vi "IR measure read.vi"(8 "error in (no error)":errorcluster, 11 "ref array":refnum<class "IR sensor.lvclass">[](array[class])) -> (0 "error out":errorcluster, 4 "output cluster":T1, 5 "Waveform Chart":T2(graph))   [LabVIEW 2019]
uses:
  IR out.ctl
  FPGA_subVIs/low level/IR sensor/IR sensor.lvclass
  <vilib>/ptbypt/NI_PtbyPt.lvlib
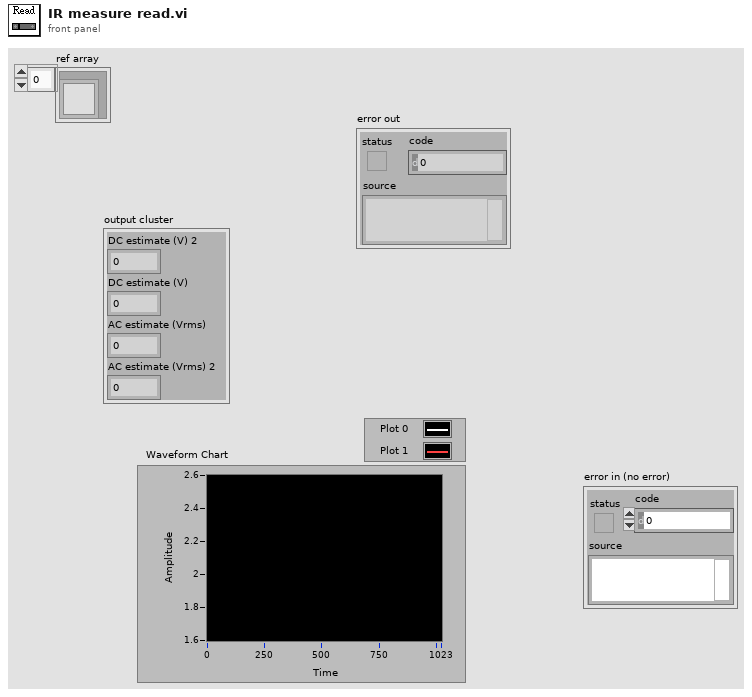
[diagram p1: front panel]
types:
  T1 = typedef "IR out.ctl" = cluster{"DC estimate (V) 2":dbl, "DC estimate (V)":dbl, "AC estimate (Vrms)":dbl, "AC estimate (Vrms) 2":dbl}
  T2 = cluster{"dbl Scaled Value":dbl, "dbl Scaled Value":dbl}
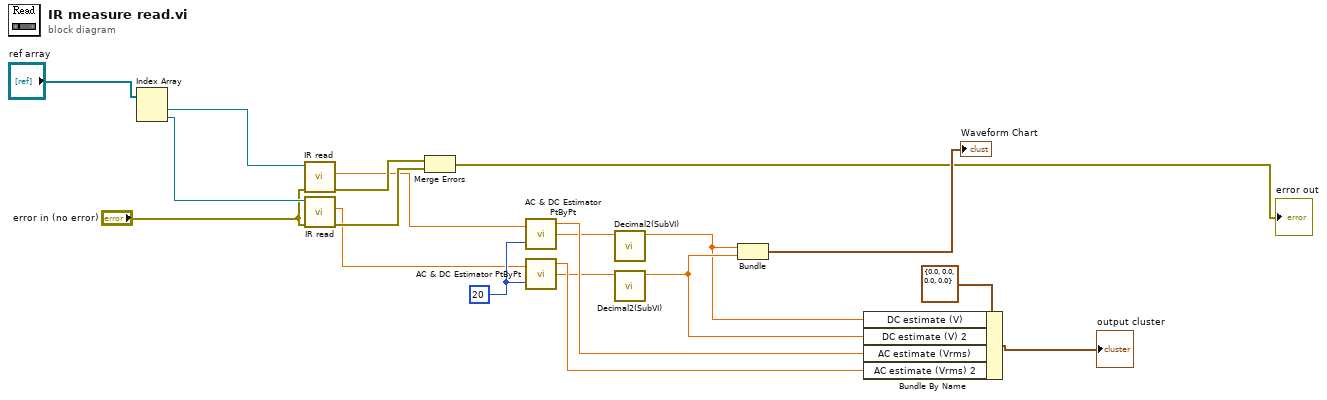
[diagram p0: block diagram]
diagram:
  w18 = 20 ("sample length")
  n1 = Index Array(array="ref array") -> (element #1=w8:refnum<class "IR sensor.lvclass">, element #2=w7:refnum<class "IR sensor.lvclass">)  [unwired: 2 in]
  n2 = call-dynamic "IR read.vi"("error in (no error)"="error in (no error)", "IR sensor in"=w8) -> ("error out"=w5:errorcluster, "IR"=w2:dbl)  [unwired: 7 in, 1 out]
  n3 = call-dynamic "IR read.vi"("error in (no error)"="error in (no error)", "IR sensor in"=w7) -> ("error out"=w4:errorcluster, "IR"=w3:dbl)  [unwired: 7 in, 1 out]
  n4 = Merge Errors(w5, w4) -> (→"error out":errorcluster)
  n5 = call <vilib>:"AC & DC Estimator PtByPt.vi"("signal"=w2, "sample length"=w18) -> ("AC estimate (Vrms)"=w15:dbl, "DC estimate (V)"=w11:dbl)  [unwired: 1 in, 1 out]
  n6 = call <vilib>:"AC & DC Estimator PtByPt.vi"("signal"=w3, "sample length"=w18) -> ("AC estimate (Vrms)"=w14:dbl, "DC estimate (V)"=w13:dbl)  [unwired: 1 in, 1 out]
  n7 = call "Decimal2(SubVI).vi"("DC estimate (V)"=w11) -> ("Numeric"=w10:dbl)  [unwired: 10 in]
  n8 = call "Decimal2(SubVI).vi"("DC estimate (V)"=w13) -> ("Numeric"=w12:dbl)  [unwired: 10 in]
  n9 = Bundle("Numeric"=w10, "Numeric"=w12) -> (→"Waveform Chart":cluster{"Numeric":dbl, "Numeric":dbl})  [unwired: 1 in]
  n10 = Bundle By Name(cluster=T1 {"DC estimate (V) 2"=0.0, "DC estimate (V)"=0.0, "AC estimate (Vrms)"=0.0, "AC estimate (Vrms) 2"=0.0} ("Cluster"), "DC estimate (V)"=w10, "DC estimate (V) 2"=w12, "AC estimate (Vrms)"=w15, "AC estimate (Vrms) 2"=w14) -> (→"output cluster":T1)
